vi "find_best_phase_2.vi"(9 "steepest slope":dbl, 10 "current phase":dbl, 11 "Array of phases":dbl[](array[numeric])) -> (1 "phase stage":bool, 2 "optimum phase":dbl, 3 "Array of phases":dbl[](array[numeric]))   [LabVIEW 2015]
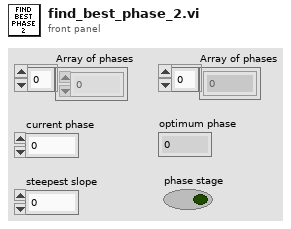
[diagram p1: front panel]
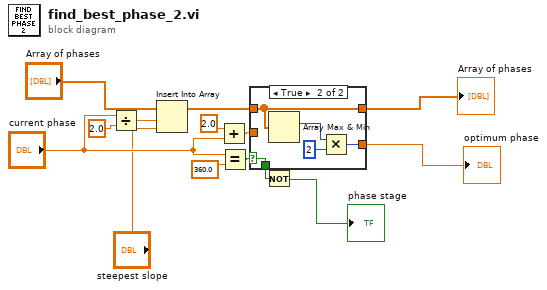
[diagram p0: block diagram]
diagram:
  n1 = Divide(x="current phase", y=2.0) -> (x/y=w11:dbl)
  n2 = Insert Into Array(array="Array of phases", index=w11, new element="steepest slope") -> (w7:dbl[])
  n3 = Add(x=2.0 ("y"), y="current phase") -> (x+y=w8:dbl)
  n4 = Equal?(x="current phase", y=360.0) -> (x = y?=w6:bool)
  n5 = case shown="True" w6 {
    selector: w6 -> [w15 w20]
    tunnel: w7 -> [w17 w21]
    tunnel: [w17 w21] -> w4
    tunnel: w8 -> [w16 _]
    tunnel: [w16 w22] -> w2
    tunnel: [w15 w20] -> w13
    frame False {
    }
    frame True {
      n6 = Array Max & Min(array=w21) -> (max index (indices)=w19:i32)  [unwired: 3 out]
      n7 = Multiply(x=w19, y=2) -> (x*y=w22:i32)
    }
  }
  "Array of phases" <- w4
  "optimum phase" <- w2
  n8 = Not(x=w13) -> (.not. x?=→"phase stage":bool)
